vi "Add Destination.vi"(8 "error in (no error)":errorcluster, 9 "Destination type (directory)":T1, 10 "Destination label":string, 11 "PPL in":refnum<class "NI_AB_API_PPL.lvclass">) -> (0 "error out":errorcluster, 3 "PPL out":refnum<class "NI_AB_API_PPL.lvclass">)   [LabVIEW 2020, in "NI_AB_API_PPL.lvclass"]
uses:
  <vilib>/AppBuilder/AB_API/PPL/NI_AB_API_PPL.lvclass
  <vilib>/AppBuilder/AB_API/common/AB_API Destination Type.ctl
  <vilib>/AppBuilder/AB_API/Targetfile/NI_AB_API_Targetfile.lvclass
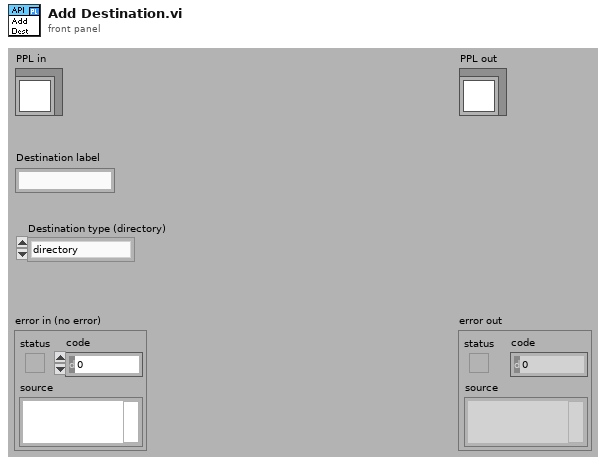
[diagram p1: front panel]
types:
  T1 = typedef "AB_API Destination Type.ctl" = enum16{"directory", "directory (preserve hierarchy)", "LLB"}
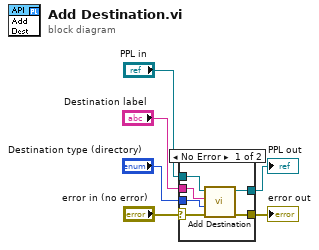
[diagram p0: block diagram]
diagram:
  n1 = case shown="No Error" "error in (no error)" {
    selector: "error in (no error)" -> [w9 w14]
    tunnel: [w7 w14] -> w4
    tunnel: [w8 w13] -> w5
    tunnel: "PPL in" -> [w12 w13]
    tunnel: "Destination label" -> [w11 _]
    tunnel: "Destination type (directory)" -> [w10 _]
    frame No Error {
      n2 = call-parent "Add Destination.vi"("error in (no error)"=w9, "Destination type (directory)"=w10, "Destination label"=w11, "Build in"=w12) -> ("error out"=w7:errorcluster, "Build out"=w8:refnum<class "NI_AB_API_PPL.lvclass">)  [unwired: 6 in]
    }
    frame Error {
    }
  }
  "error out" <- w4
  "PPL out" <- w5
